vi "ma_SML Averaging (complex input).vi"(3 "reset?":bool, 4 "averaging settings":T1, 5 "x":cdb[](array[numeric]) format="%.2f") -> (0 "data ready?":bool, 1 "averaged sofar":dbl, 2 "y":cdb[](array[numeric]) format="%.2f")   [LabVIEW 2020, in "NI_MAPro.lvlib"]
uses:
  NI_MAPro.lvlib
  ma_sml_Averaging Settings.ctl
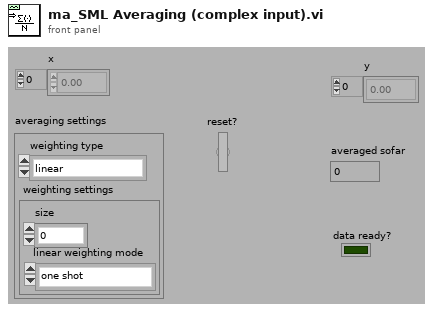
[diagram p1: front panel]
types:
  T1 = typedef "NI_MAPro.lvlib/ma_sml_Averaging Settings.ctl" = cluster{"weighting type":enum16{"linear", "exponential"}, "weighting settings":cluster{"size":dbl, "linear weighting mode":enum16{"one shot", "auto restart one shot", "moving average", "continuous"}}}
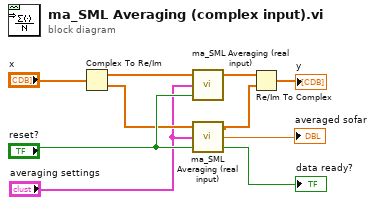
[diagram p0: block diagram]
diagram:
  n1 = Complex To Re/Im(x + iy="x") -> (x=w4:dbl[], y=w3:dbl[])
  n2 = call "ma_SML Averaging (real input).vi"("reset?"="reset?", "averaging settings"="averaging settings", "x"=w4) -> ("y"=w9:dbl[])  [unwired: 2 out]
  n3 = call "ma_SML Averaging (real input).vi"("reset?"="reset?", "averaging settings"="averaging settings", "x"=w3) -> ("data ready?"=→"data ready?":bool, "averaged sofar"=→"averaged sofar":dbl, "y"=w8:dbl[])
  n4 = Re/Im To Complex(1:w8, 2:w9) -> (0:→"y":cdb[])
